vi "VCS Get Recorder Parameter.vi"(0 "axis in":cluster{"keyHandle":u32, "nodeId":u16}={"keyHandle"=0, "nodeId"=1}, 11 "error in (no error)":errorcluster) -> (4 "axis out":cluster{"keyHandle":u32, "nodeId":u16}={"keyHandle"=0, "nodeId"=1}, 6 "recorder parameter":T1, 15 "error out":errorcluster)   [LabVIEW 2010]
doc: "<B>VCS_GetRecorderParameter</B> reads parameters for data recorder."
uses:
  Resources/EposCmd.dll
  Resources/EposCmd64.dll
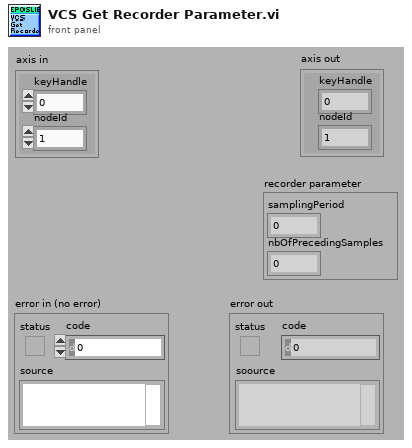
[diagram p1: front panel]
types:
  T1 = cluster{"samplingPeriod":u16, "nbOfPrecedingSamples":u16}
  T2 = cluster{"pSamplingPeriod":u16, "pNbOfPrecedingSamples":u16}
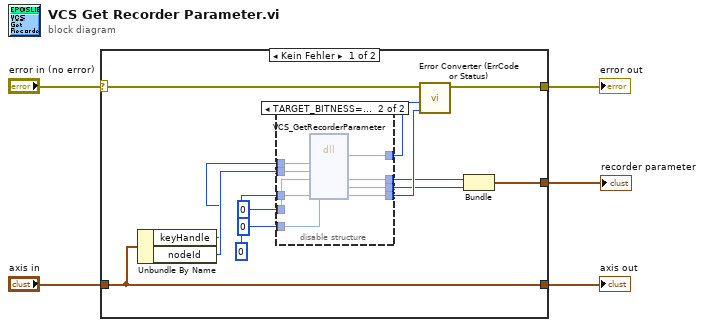
[diagram p0: block diagram]
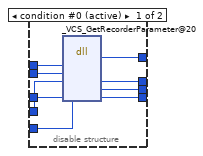
[diagram p2: hidden frame]
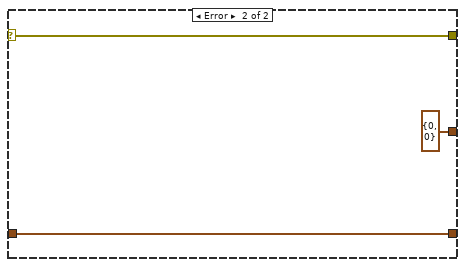
[diagram p3: hidden frame]
diagram:
  n1 = case shown="Kein Fehler" "error in (no error)" {
    selector: "error in (no error)" -> [w16 w38]
    tunnel: "axis in" -> [w18 w39]
    tunnel: [w18 w39] -> w4
    tunnel: [w17 w38] -> w3
    tunnel: [w8 T2 {"pSamplingPeriod"=0, "pNbOfPrecedingSamples"=0}] -> w1
    frame No Error {
      n2 = Unbundle By Name(w18) -> ("keyHandle"=w13:u32, "nodeId"=w14:u16)
      n3 = disable-structure shown="TARGET_BITNESS==64" {
        disable-tunnel: u32 0 ("pErrorCode") -> [w27 w36]
        disable-tunnel: w14 -> [w26 w35]
        disable-tunnel: w13 -> [w25 w34]
        disable-tunnel: [w24 w33] -> w12
        disable-tunnel: [w23 w32] -> w11
        disable-tunnel: [w22 w31] -> w10
        disable-tunnel: [w21 w30] -> w9
        disable-tunnel: u16 0 ("pSamplingPeriod") -> [w20 w29]
        disable-tunnel: u16 0 ("pNbOfPrecedingSamples") -> [w19 w28]
        frame condition #0 (active) {
          n4 = dll-call lib="C:/Sources/LabView/maxon EPOS/Resources/EposCmd.*" fn="_VCS_GetRecorderParameter@20"("KeyHandle"=w25, "NodeId"=w26, "pSamplingPeriod"=w20, "pNbOfPrecedingSamples"=w19, "pErrorCode"=w27) -> (w24:i32, "pSamplingPeriod"=w22:u16, "pNbOfPrecedingSamples"=w21:u16, "pErrorCode"=w23:u32)  [unwired: 5 in, 2 out]
        }
        frame condition #1 {
          n5 = dll-call lib="C:/setup/Resources/EposCmd64.*" fn="VCS_GetRecorderParameter" ("EposCmd.dll:_VCS_GetRecorderParameter@20")("KeyHandle"=w34, "NodeId"=w35, "pSamplingPeriod"=w29, "pNbOfPrecedingSamples"=w28, "pErrorCode"=w36) -> ("Rückgabetyp"=w33:i32, "pSamplingPeriod"=w31:u16, "pNbOfPrecedingSamples"=w30:u16, "pErrorCode"=w32:u32)  [unwired: 5 in, 2 out]
        }
      }
      n6 = call "Error Converter (ErrCode or Status).vi"("error code"=w11, "return type"=w12, "error in (no error)"=w16) -> ("error out"=w17:errorcluster)  [unwired: 7 in]
      n7 = Bundle("pSamplingPeriod"=w10, "pNbOfPrecedingSamples"=w9) -> (w8:T2)  [unwired: 1 in]
    }
    frame Error {
    }
  }
  "error out" <- w3
  "axis out" <- w4
  "recorder parameter" <- w1
